vi "Arcade Drive with Joysticks.vi"(10 "Y Axis":dbl, 11 "X Axis":dbl) -> (2 "Speed":dbl, 3 "Turn":dbl)   [LabVIEW 2016]
uses:
  <vilib>/Rock Robotics/Network Tables/NT Read Number.vi
  <vilib>/Rock Robotics/Network Tables/NT Read Boolean.vi
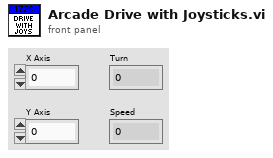
[diagram p1: front panel]
types:
  T1 = cluster{"Numeric":dbl, "Numeric":dbl, "Numeric":dbl}
  T2 = cluster{"Numeric":dbl, "Numeric":dbl, "Boolean":bool, "Numeric":dbl}
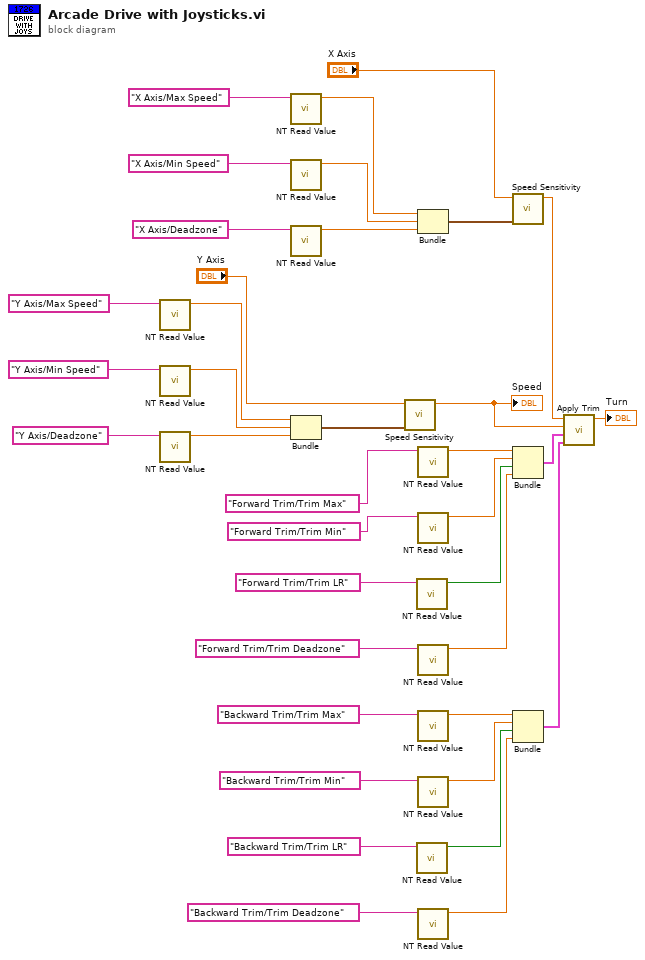
[diagram p0: block diagram]
diagram:
  n1 = call-poly <vilib>:"NT Read Value.vi"("Name"="Y Axis/Max Speed") -> ("Numeric"=w9:dbl)  [unwired: 9 in, 1 out]
  n2 = call-poly <vilib>:"NT Read Value.vi"("Name"="Y Axis/Min Speed") -> ("Numeric"=w8:dbl)  [unwired: 9 in, 1 out]
  n3 = call-poly <vilib>:"NT Read Value.vi"("Name"="Y Axis/Deadzone") -> ("Numeric"=w7:dbl)  [unwired: 9 in, 1 out]
  n4 = call-poly <vilib>:"NT Read Value.vi"("Name"="X Axis/Max Speed") -> ("Numeric"=w4:dbl)  [unwired: 9 in, 1 out]
  n5 = call-poly <vilib>:"NT Read Value.vi"("Name"="X Axis/Min Speed") -> ("Numeric"=w3:dbl)  [unwired: 9 in, 1 out]
  n6 = call-poly <vilib>:"NT Read Value.vi"("Name"="X Axis/Deadzone") -> ("Numeric"=w2:dbl)  [unwired: 9 in, 1 out]
  n7 = Bundle("Numeric"=w9, "Numeric"=w8, "Numeric"=w7) -> (w6:T1)  [unwired: 1 in]
  n8 = call "Speed Sensitivity.vi"("Tuning"=w6, "Input"="Y Axis") -> ("Output"=w37:dbl)  [unwired: 9 in]
  "Speed" <- w37
  n9 = call-poly <vilib>:"NT Read Value.vi"("Name"="Forward Trim/Trim LR") -> ("Boolean"=w19:bool)  [unwired: 9 in, 1 out]
  n10 = call-poly <vilib>:"NT Read Value.vi"("Name"="Backward Trim/Trim LR") -> ("Boolean"=w30:bool)  [unwired: 9 in, 1 out]
  n11 = Bundle("Numeric"=w4, "Numeric"=w3, "Numeric"=w2) -> (w1:T1)  [unwired: 1 in]
  n12 = call-poly <vilib>:"NT Read Value.vi"("Name"="Forward Trim/Trim Max") -> ("Numeric"=w17:dbl)  [unwired: 9 in, 1 out]
  n13 = call-poly <vilib>:"NT Read Value.vi"("Name"="Forward Trim/Trim Min") -> ("Numeric"=w18:dbl)  [unwired: 9 in, 1 out]
  n14 = call-poly <vilib>:"NT Read Value.vi"("Name"="Forward Trim/Trim Deadzone") -> ("Numeric"=w16:dbl)  [unwired: 9 in, 1 out]
  n15 = call-poly <vilib>:"NT Read Value.vi"("Name"="Backward Trim/Trim Max") -> ("Numeric"=w28:dbl)  [unwired: 9 in, 1 out]
  n16 = call-poly <vilib>:"NT Read Value.vi"("Name"="Backward Trim/Trim Min") -> ("Numeric"=w29:dbl)  [unwired: 9 in, 1 out]
  n17 = call-poly <vilib>:"NT Read Value.vi"("Name"="Backward Trim/Trim Deadzone") -> ("Numeric"=w27:dbl)  [unwired: 9 in, 1 out]
  n18 = call "Speed Sensitivity.vi"("Tuning"=w1, "Input"="X Axis") -> ("Output"=w21:dbl)  [unwired: 9 in]
  n19 = Bundle("Numeric"=w17, "Numeric"=w18, "Boolean"=w19, "Numeric"=w16) -> (w22:T2)  [unwired: 1 in]
  n20 = Bundle("Numeric"=w28, "Numeric"=w29, "Boolean"=w30, "Numeric"=w27) -> (w32:T2)  [unwired: 1 in]
  n21 = call "Apply Trim.vi"("Backwards Tuning"=w32, "Forward Tuning"=w22, "Speed"=w37, "Turn"=w21) -> ("Trimmed Turn"=→"Turn":dbl)  [unwired: 7 in]
